vi "Merge Error.vi"(10 "Error":errorcluster, 11 "jettl Actor in":refnum<class "jettl Actor.lvclass">) -> (3 "jettl Actor out":refnum<class "jettl Actor.lvclass">)   [LabVIEW 2021, in "jettl.lvlib" / "Temporary Actor.lvlib" / "jettl Actor.lvclass"]
uses:
  jettl Actor.lvclass
  jettl Actor.lvclass/jettl Actor.ctl
  State.ctl
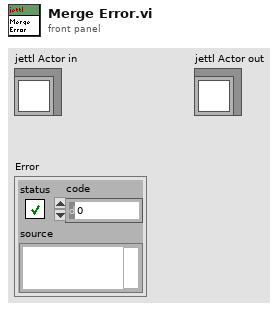
[diagram p1: front panel]
types:
  T1 = typedef "jettl.lvlib/Temporary Actor.lvlib/jettl Actor.lvclass/State.ctl" = enum16{"Nominal", "Teardown", "Error"}
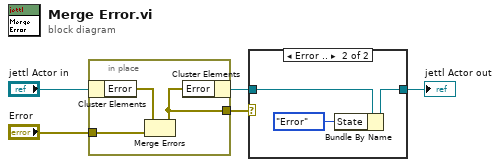
[diagram p0: block diagram]
diagram:
  n1 = in-place {
    in-place-border: "Error" -> [w7]
    in-place-border: [w6] -> w1
    n2 = in-place-cluster #1("jettl Actor in") -> ("Error"=w8:errorcluster)
    n3 = Merge Errors(w8, w7) -> (w6:errorcluster)
    n4 = in-place-cluster #1("Error"=w6) -> (w3:refnum<class "jettl Actor.lvclass">)
  }
  n5 = case shown="Error .." w1 {
    tunnel: [w9 w11] -> w2
    tunnel: w3 -> [w9 w12]
    frame No Error {
    }
    frame Error {
      n6 = Bundle By Name(cluster=w12, "State"=State."Error") -> (w11:refnum<class "jettl Actor.lvclass">)
    }
  }
  "jettl Actor out" <- w2
